vi "Constant Array Size Sha-1.vi"(11 "Message In as Byte Array":u8[](array[numeric])=[97, 0, 0, 0, 0, 0, 0, 0, 0, 0, 0, 0, 0, 0, 0, 0, 0, 0, 0, 0, 0, 0, 0, 0, 0, 0, 0, 0, 0, 0, 0, 0, 0, 0, 0, 0, 0, 0, 0, 0, 0, 0, 0, 0, 0, 0, 0, 0, 0, 0, 0, 0, 0, 0, 0, 0, 0, 0, 0, 0, 0, 0, 0, 0, 0, 0, 0, 0, 0, 0, 0, 0, 0, 0, 0, 0, 0, 0, 0, 0, 0, 0, 0, 0, 0, 0, 0, 0, 0, 0, 0, 0, 0, 0, 0, 0, 0, 0, 0, 0, 0, 0, 0, 0, 0, 0, 0, 0, 0, 0, 0, 0, 0, 0, 0, 0, 0, 0, 0]) -> (3 "Digest":u8[](array[numeric]) format="%x")   [LabVIEW 2014]
uses:
  <vilib>/rvi/DataTransferAndStorage/Container/Common/niFpgaContainerGetUniqueNameForEmu.vi
  <vilib>/rvi/DataTransferAndStorage/Container/Common/niFpgaContainerSetEmuInfo.vi
  <vilib>/rvi/eio/common/nirviEmuReportErrorAndStop.vi
  <vilib>/rvi/DataTransferAndStorage/Container/Common/niFpgaContainerExecOnDevCompGetState.vi
  <vilib>/rvi/Emulation/niFpgaEmulationIsFPGAContextNoSignature.vi
  <vilib>/rvi/Emulation/niFpgaProcessEmulError.vi
  <vilib>/rvi/Emulation/niFpgaSctlEmulationGetInTimedLoop.vi
  <vilib>/rvi/errors/nirviReportUnexpectedCaseInternalError (U32).vi
  <vilib>/rvi/Memory/Memory_Emulation/niFpgaMemoryEmulationCacheClearOnFirstRun.vi
  <vilib>/rvi/Memory/Memory_Emulation/nirvimemoryEmulationManagerCache_MakeExclusive.vi
  <vilib>/rvi/Memory/Memory_Emulation/niFpgaMemoryEmulationValidateCache.vi
  <vilib>/rvi/Memory/Memory_Emulation/nirvimemoryEmulationManagerCache_InsertValue.vi
  <vilib>/Utility/error.llb/Clear Errors.vi
  <vilib>/rvi/Memory/Memory_Emulation/nirvimemoryEmulationManagerCache_ReleaseExclusive.vi
  <vilib>/rvi/Memory/Memory_Emulation/nirvimemoryEmulationManagerCache_GetValue.vi
  <vilib>/rvi/Memory/Memory_Emulation/nirvimemoryEmulationManagerCache_SetValue.vi
  <vilib>/rvi/Emulation/niFpgaSctlEmulationResourceMgr.vi
  <vilib>/rvi/LocalResourceManager/LocalResourceManager.xnode
  <vilib>/rvi/DataTransferAndStorage/Container/XNode/niFpgaContainer.xnode
  <vilib>/rvi/Memory/Memory_Emulation/niFpgaMemoryEmulationRefIn.vi
panel:
  out "x-y":u32
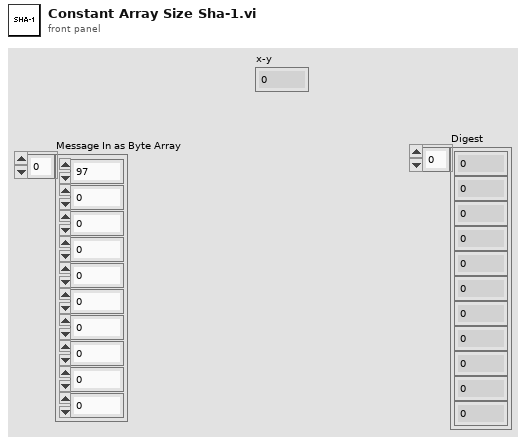
[diagram p1: front panel]
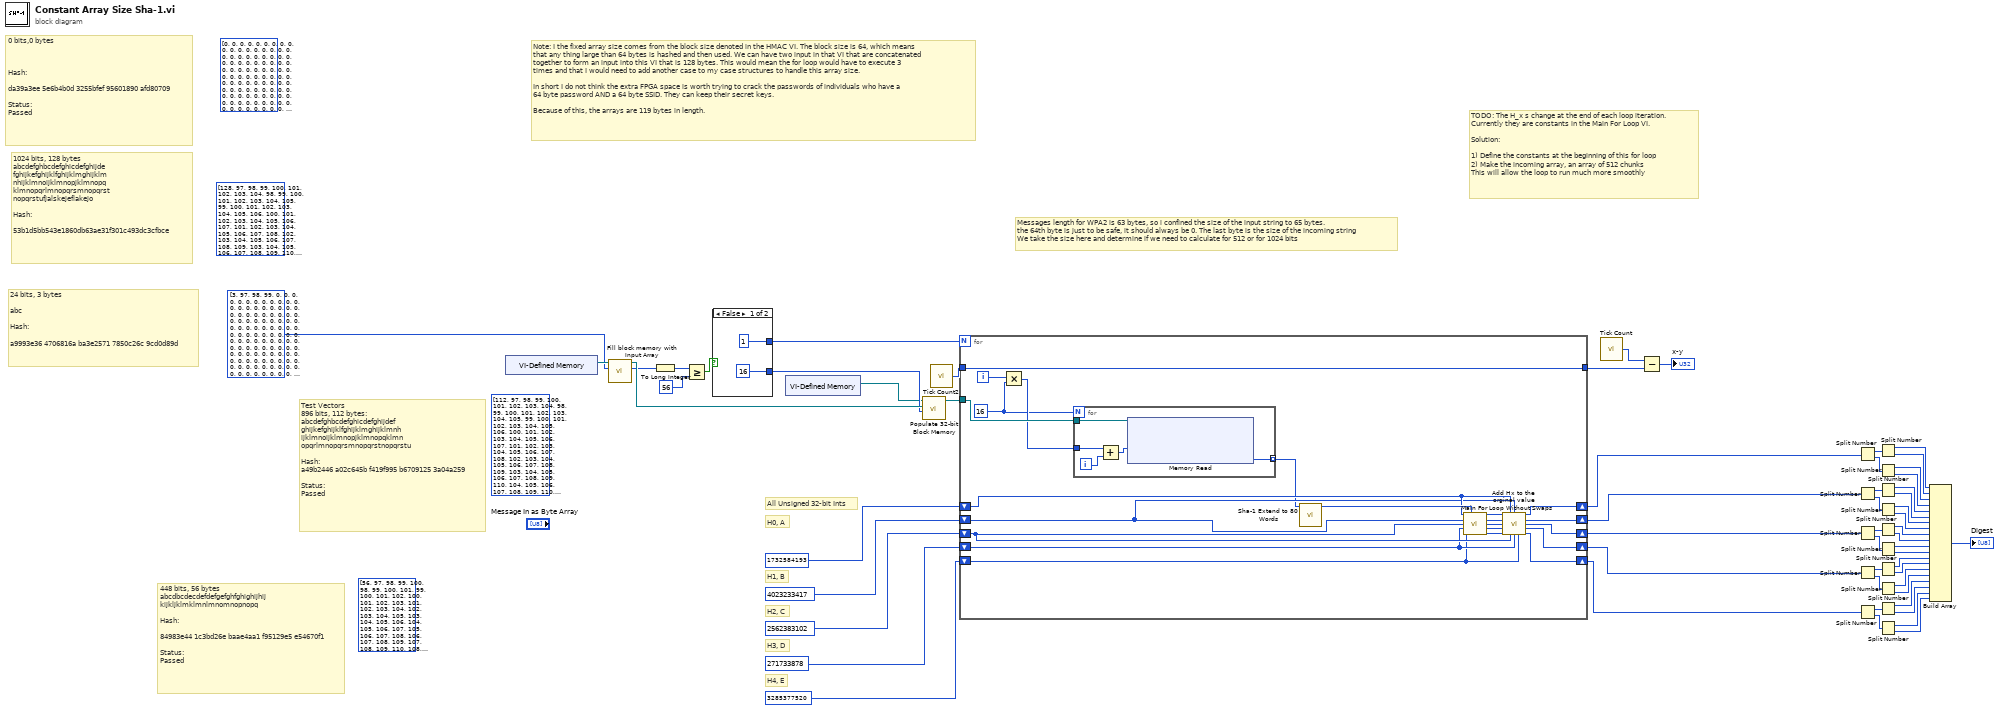
[diagram p0: block diagram]
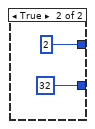
[diagram p2: hidden frame]
diagram:
  (unwired) u8[] [128, 97, 98, 99, 100, 101, 102, 103, 104, 98, 99, 100, 101, 102, 103, 104, 105, 99, 100, 101, 102, 103, 104, 105, 106, 100, 101, 102, 103, 104, 105, 106, 107, 101, 102, 103, 104, 105, 106, 107, 108, 102, 103, 104, 105, 106, 107, 108, 109, 103, 104, 105, 106, 107, 108, 109, 110, 104, 105, 106, 107, 108, 109, 110, 111, 105, 106, 107, 108, 109, 110, 111, 112, 106, 107, 108, 109, 110, 111, 112, 113, 107, 108, 109, 110, 111, 112, 113, 114, 108, 109, 110, 111, 112, 113, 114, 115, 109, 110, 111, 112, 113, 114, 115, 116, 110, 111, 112, 113, 114, 115, 116, 117, 102, 106, 97, 108, 115, 107] ("appended array")
  (unwired) u8[] [0, 0, 0, 0, 0, 0, 0, 0, 0, 0, 0, 0, 0, 0, 0, 0, 0, 0, 0, 0, 0, 0, 0, 0, 0, 0, 0, 0, 0, 0, 0, 0, 0, 0, 0, 0, 0, 0, 0, 0, 0, 0, 0, 0, 0, 0, 0, 0, 0, 0, 0, 0, 0, 0, 0, 0, 0, 0, 0, 0, 0, 0, 0, 0, 0, 0, 0, 0, 0, 0, 0, 0, 0, 0, 0, 0, 0, 0, 0, 0, 0, 0, 0, 0, 0, 0, 0, 0, 0, 0, 0, 0, 0, 0, 0, 0, 0, 0, 0, 0, 0, 0, 0, 0, 0, 0, 0, 0, 0, 0, 0, 0, 0, 0, 0, 0, 0, 0, 0] ("appended array")
  (unwired) u8[] [56, 97, 98, 99, 100, 98, 99, 100, 101, 99, 100, 101, 102, 100, 101, 102, 103, 101, 102, 103, 104, 102, 103, 104, 105, 103, 104, 105, 106, 104, 105, 106, 107, 105, 106, 107, 108, 106, 107, 108, 109, 107, 108, 109, 110, 108, 109, 110, 111, 109, 110, 111, 112, 110, 111, 112, 113, 0, 0, 0, 0, 0, 0, 0, 0, 0, 0, 0, 0, 0, 0, 0, 0, 0, 0, 0, 0, 0, 0, 0, 0, 0, 0, 0, 0, 0, 0, 0, 0, 0, 0, 0, 0, 0, 0, 0, 0, 0, 0, 0, 0, 0, 0, 0, 0, 0, 0, 0, 0, 0, 0, 0, 0, 0, 0, 0, 0, 0, 0] ("appended array")
  (unwired) u8[] [112, 97, 98, 99, 100, 101, 102, 103, 104, 98, 99, 100, 101, 102, 103, 104, 105, 99, 100, 101, 102, 103, 104, 105, 106, 100, 101, 102, 103, 104, 105, 106, 107, 101, 102, 103, 104, 105, 106, 107, 108, 102, 103, 104, 105, 106, 107, 108, 109, 103, 104, 105, 106, 107, 108, 109, 110, 104, 105, 106, 107, 108, 109, 110, 111, 105, 106, 107, 108, 109, 110, 111, 112, 106, 107, 108, 109, 110, 111, 112, 113, 107, 108, 109, 110, 111, 112, 113, 114, 108, 109, 110, 111, 112, 113, 114, 115, 109, 110, 111, 112, 113, 114, 115, 116, 110, 111, 112, 113, 114, 115, 116, 117, 0, 0, 0, 0, 0, 0] ("Test Vector 2")
  # "Note: I the fixed array size comes from the block size denoted in the HMAC VI. The block size is 64, which means\nthat any thing large than 64 bytes is hashed and then used. We can have two input in that VI that are concatenated \ntogether to form an input into this VI that is 128 bytes. This would mean the for loop would have to execute 3 \ntimes and that I would need to add another case to my case structures to handle this array size. \n\nIn short I do not think the extra FPGA space is worth trying to crack the passwords of individuals who have a\n64 byte password AND a 64 byte SSID. They can keep their secret keys. \n\nBecause of this, the arrays are 119 bytes in length."
  # "0 bits,0 bytes\n\n\n\nHash:\n\nda39a3ee 5e6b4b0d 3255bfef 95601890 afd80709\n\nStatus:\nPassed"
  # "24 bits, 3 bytes\n\nabc\n\nHash:\n\na9993e36 4706816a ba3e2571 7850c26c 9cd0d89d"
  # "448 bits, 56 bytes\nabcdbcdecdefdefgefghfghighijhij\nkijkljklmklmnlmnomnopnopq\n\nHash:\n\n84983e44 1c3bd26e baae4aa1 f95129e5 e54670f1\n\nStatus: \nPassed"
  # "1024 bits, 128 bytes\nabcdefghbcdefghicdefghijde\nfghijkefghijklfghijklmghijklm\nnhijklmnoijklmnopjklmnopq\nklmnopqrlmnopqrsmnopqrst\nnopqrstufjalskejeflakejo\n\nHash:\n\n53b1d5bb543e1860db63ae31f301c493dc3cfbce"
  # "Test Vectors\n896 bits, 112 bytes:\nabcdefghbcdefghicdefghijdef\nghijkefghijklfghijklmghijklmnh\nijklmnoijklmnopjklmnopqklmn\nopqrlmnopqrsmnopqrstnopqrstu\n\nHash:\na49b2446 a02c645b f419f995 b6709125 3a04a259\n\nStatus:\nPassed"
  # "All Unsigned 32-bit Ints"
  # "H0, A"
  # "H3, D"
  # "H4, E"
  # "H2, C"
  # "H1, B"
  # "TODO: The H_x s change at the end of each loop iteration. \nCurrently they are constants in the Main For Loop VI. \n\nSolution:\n\n1) Define the constants at the beginning of this for loop\n2) Make the incoming array, an array of 512 chunks\nThis will allow the loop to run much more smoothly"
  # "Messages length for WPA2 is 63 bytes, so i confined the size of the input string to 65 bytes. \nthe 64th byte is just to be safe, it should always be 0. The last byte is the size of the incoming string\nWe take the size here and determine if we need to calculate for 512 or for 1024 bits"
  n1 = xnode "VI-Defined Memory"() -> ("Memory Out"=w12:refnum<k21>)
  n2 = call "Fill block memory with Input Array.vi"("Message In"=u8[] [3, 97, 98, 99, 0, 0, 0, 0, 0, 0, 0, 0, 0, 0, 0, 0, 0, 0, 0, 0, 0, 0, 0, 0, 0, 0, 0, 0, 0, 0, 0, 0, 0, 0, 0, 0, 0, 0, 0, 0, 0, 0, 0, 0, 0, 0, 0, 0, 0, 0, 0, 0, 0, 0, 0, 0, 0, 0, 0, 0, 0, 0, 0, 0, 0, 0, 0, 0, 0, 0, 0, 0, 0, 0, 0, 0, 0, 0, 0, 0, 0, 0, 0, 0, 0, 0, 0, 0, 0, 0, 0, 0, 0, 0, 0, 0, 0, 0, 0, 0, 0, 0, 0, 0, 0, 0, 0, 0, 0, 0, 0, 0, 0, 0, 0, 0, 0, 0, 0] ("appended array"), "Block Memory Reference In"=w12) -> ("Array Length"=w7:u8, "Block Memory Reference Out"=w11:refnum<k21>)  [unwired: 8 in]
  n3 = To Long Integer(number=w7) -> (32bit integer=w6:i32)
  n4 = Greater Or Equal?(x=w6, y=56) -> (x >= y?=w14:bool)
  n5 = case shown="False" w14 {
    tunnel: [1 2] -> w13
    tunnel: [16 32] -> w10
    frame False {
    }
    frame True {
    }
  }
  n6 = xnode "VI-Defined Memory"() -> ("Memory Out"=w9:refnum<k21>)
  n7 = call "Populate 32-bit Block Memory.vi"("Number of U32 words in Array"=w10, "Boolean array Block Mem in"=w11, "U32 Block Mem in"=w9) -> ("U32 Block mem Out"=w8:refnum<k21>)  [unwired: 8 in]
  n8 = call "Tick Count2"() -> ("Tick Count(Ticks)"=w4:u32)
  n9 = for {
    N: w13 -> [_]
    shift-right: [w77] -> w51
    shift-left: u32 1732584193 -> [w71]
    shift-right: [w76] -> w38
    shift-left: u32 4023233417 -> [w70]
    shift-right: [w75] -> w29
    shift-left: u32 2562383102 -> [w69]
    shift-right: [w74] -> w28
    shift-left: u32 271733878 -> [w68]
    shift-right: [w73] -> w25
    shift-left: u32 3285377520 -> [w67]
    tunnel: w8 -> [w65]
    tunnel: w4 -> [w61]
    tunnel: [w61] -> w3
    i -> [w66]
    w63 = 16 ("length")
    n10 = Multiply(x=w66, y=w63) -> (x*y=w64:i32)
    n11 = for {
      N: w63 -> [_]
      tunnel: w65 -> [w87]
      tunnel: w64 -> [w85]
      tunnel: [w83] -> w62 mode=indexing
      i -> [w86]
      n12 = Add(x=w85, y=w86) -> (x+y=w84:i32)
      n13 = xnode ("Memory Read")("Address"=w84, "Memory In"=w87) -> ("Data"=w83:u32)  [unwired: 1 out]
    }
    n14 = call "Sha-1 Extend to 80 Words.vi"("16 32-bit Words In"=w62) -> ("80 32 Bit Words Out"=w72:u32[])  [unwired: 10 in]
    n15 = call "Main For Loop Without Swaps.vi"("A"=w71, "80 32-bit Words"=w72, "B"=w70, "C"=w69, "D"=w68, "E"=w67) -> ("A Out"=w82:u32, "B Out"=w81:u32, "C Out"=w80:u32, "D Out"=w79:u32, "E Out"=w78:u32)  [unwired: 5 in]
    n16 = call "Add Hx to the orginal value.vi"("A Out"=w82, "H0 In"=w71, "H1 In"=w70, "B Out"=w81, "C Out"=w80, "D Out"=w79, "E Out"=w78, "H2 In"=w69, "H3 In"=w68, "H4 In"=w67) -> ("H0"=w77:u32, "H1"=w76:u32, "H2"=w75:u32, "H3"=w74:u32, "H4"=w73:u32)  [unwired: 1 in]
  }
  n17 = call "Tick Count"() -> ("Tick Count(Ticks)"=w2:u32)
  n18 = Subtract(x=w2, y=w3) -> (x-y=→"x-y":u32)
  n19 = Split Number(x=w51) -> (hi(x)=w50:u16, lo(x)=w49:u16)
  n20 = Split Number(x=w38) -> (hi(x)=w43:u16, lo(x)=w44:u16)
  n21 = Split Number(x=w29) -> (hi(x)=w36:u16, lo(x)=w37:u16)
  n22 = Split Number(x=w28) -> (hi(x)=w30:u16, lo(x)=w31:u16)
  n23 = Split Number(x=w25) -> (hi(x)=w27:u16, lo(x)=w26:u16)
  n24 = Split Number(x=w50) -> (hi(x)=w48:u8, lo(x)=w47:u8)
  n25 = Split Number(x=w49) -> (hi(x)=w46:u8, lo(x)=w45:u8)
  n26 = Split Number(x=w43) -> (hi(x)=w42:u8, lo(x)=w41:u8)
  n27 = Split Number(x=w44) -> (hi(x)=w40:u8, lo(x)=w39:u8)
  n28 = Split Number(x=w36) -> (hi(x)=w35:u8, lo(x)=w34:u8)
  n29 = Split Number(x=w37) -> (hi(x)=w33:u8, lo(x)=w32:u8)
  n30 = Split Number(x=w30) -> (hi(x)=w24:u8, lo(x)=w23:u8)
  n31 = Split Number(x=w31) -> (hi(x)=w22:u8, lo(x)=w21:u8)
  n32 = Split Number(x=w27) -> (hi(x)=w20:u8, lo(x)=w19:u8)
  n33 = Split Number(x=w26) -> (hi(x)=w18:u8, lo(x)=w17:u8)
  n34 = Build Array(w48, w47, w46, w45, w42, w41, w40, w39, w35, w34, w33, w32, w24, w23, w22, w21, w20, w19, w18, w17) -> (→"Digest":u8[])
